vi "get subscriptions queue.vi"(8 "error in":errorcluster {"code" format="Error %.0f"}, 11 "NATS Client in":refnum<class "NATS Client.lvclass">) -> (0 "error out":errorcluster {"code" format="Error %.0f"}, 2 "subscriptions queue":refnum<queue>, 3 "NATS Client out":refnum<class "NATS Client.lvclass">)   [LabVIEW 2024, in "NATS Client.lvlib" / "NATS Client.lvclass"]
uses:
  NATS Client.lvclass
  subscription queue.ctl
  subscription actions.ctl
  NATS Subscription/NATS Subscription.lvclass
  NATS Client.lvclass/NATS Client.ctl
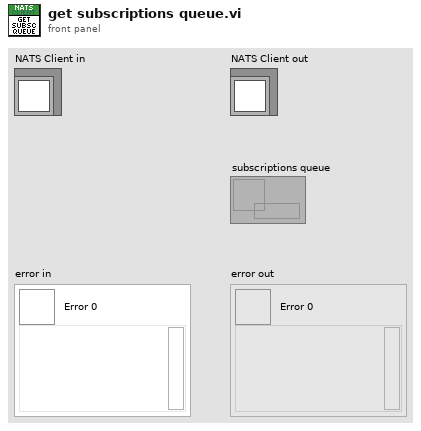
[diagram p1: front panel]
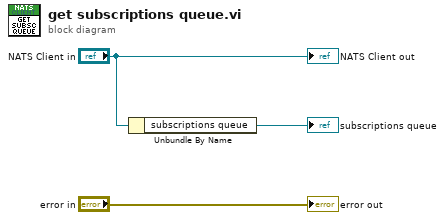
[diagram p0: block diagram]
diagram:
  n1 = Unbundle By Name("NATS Client in") -> ("subscriptions queue"=→"subscriptions queue":refnum<queue>)
  "error out" <- "error in"
  "NATS Client out" <- "NATS Client in"
